vi "Get Transfer Group by ID.vi"(8 "error in (no error)":errorcluster, 10 "Transfer Group id":i32, 11 "Transceiver Thread in":refnum<class "Transceiver Thread.lvclass">) -> (0 "error out":errorcluster, 2 "Transfer Group":refnum<class "Transfer Group.lvclass">, 3 "Transceiver Thread out":refnum<class "Transceiver Thread.lvclass">)   [LabVIEW 2017, in "DSF Core.lvlib" / "Transceiver Thread.lvclass"]
uses:
  Transceiver Thread.lvclass
  Transfer/Transfer Group.lvclass
  Transceiver Thread.lvclass/Transceiver Thread.ctl
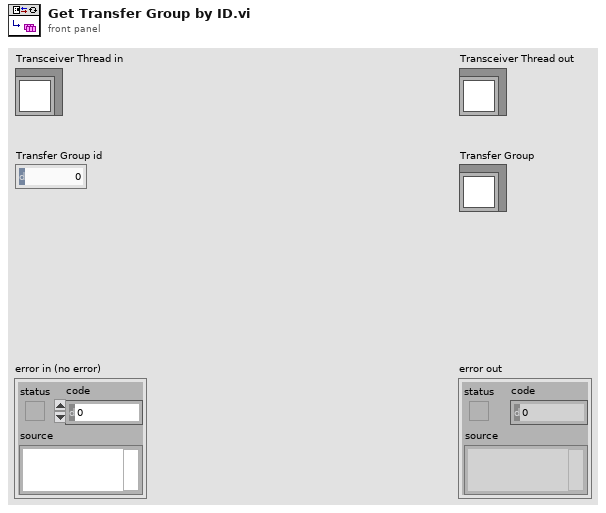
[diagram p1: front panel]
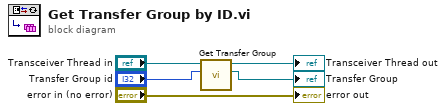
[diagram p0: block diagram]
diagram:
  n1 = call "Get Transfer Group.vi"("index"="Transfer Group id", "Transceiver Thread in"="Transceiver Thread in") -> ("Transfer Group"=→"Transfer Group":refnum<class "Transfer Group.lvclass">, "Transceiver Thread out"=→"Transceiver Thread out":refnum<class "Transceiver Thread.lvclass">)  [unwired: 8 in]
  "error out" <- "error in (no error)"
